vi "CHOOSE.vi"() -> (0 "Numeric":i32)   [LabVIEW 2014]
panel:
  in  "選擇難度":cluster{bool, bool}
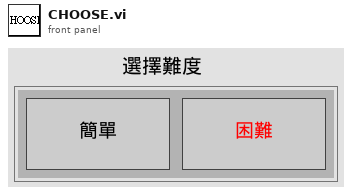
[diagram p1: front panel]
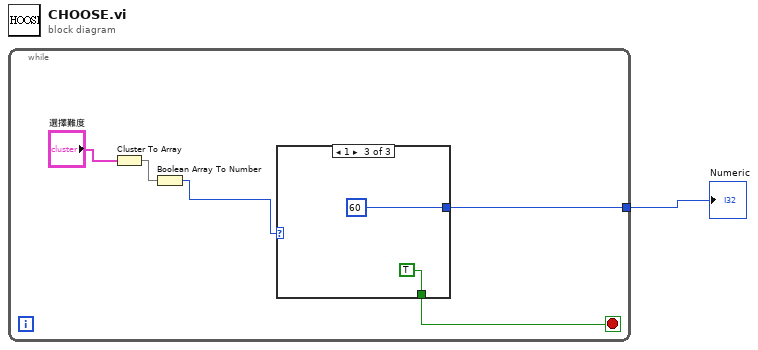
[diagram p0: block diagram]
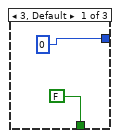
[diagram p2: hidden frame]
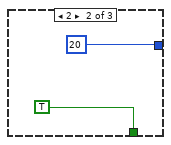
[diagram p3: hidden frame]
diagram:
  n1 = while {
    tunnel: [w2] -> w1
    stop <- w5 stop-if-true
    n2 = Cluster To Array(cluster="選擇難度") -> (array=w4:bool[])
    n3 = Boolean Array To Number(Boolean array=w4) -> (number=w3:u32)
    n4 = case shown="1" w3 {
      tunnel: [FALSE TRUE TRUE] -> w5
      tunnel: [0 20 60] -> w2
      frame 3, Default {
      }
      frame 2 {
      }
      frame 1 {
      }
    }
  }
  "Numeric" <- w1
